vi "niDTS Comm to Comm Telnet.vi"(7 "Comm Handle":T1, 9 "error in (no error)":errorcluster) -> (8 "Comm String Handle Out":T2, 10 "error out":errorcluster)   [LabVIEW 2014, in "niDTS CommLib.lvlib"]
doc: "This sends the Command concatenated with the Args over the String Interface.\n\nInputs:\n* Command (Required): This is the command to be sent.\n* Args (Optional): Any arguments to be concatenated with the command.\n\nOutputs:\n* Response: Any data returned from the interface. Note that no data wil be returned if the flag Read Enabled is set to FALSE."
uses:
  niDTS CommLib.lvlib
  Includes/niDTS Comm String INC Handle.ctl
  Objects/String_class/niDTS Comm String.lvclass
  Framework/Comm/Includes/niDTS Comm INC Handle.ctl
  Framework/Comm/Objects/BASE_class/niDTS Comm.lvclass
  Includes/niDTS Comm Telnet INC Handle.ctl
  Objects/Telnet_class/niDTS Comm Telnet.lvclass
  Framework/niDTS Framework.lvlib
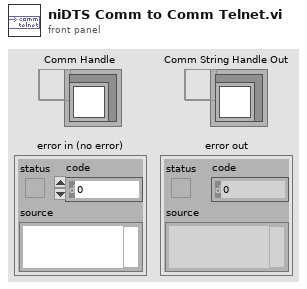
[diagram p1: front panel]
types:
  T1 = typedef "niDTS Framework.lvlib/niDTS Comm INC Handle.ctl" = refnum<data-value>
  T2 = typedef "niDTS CommLib.lvlib/niDTS Comm String INC Handle.ctl" = refnum<data-value>
  T3 = typedef "niDTS CommLib.lvlib/niDTS Comm Telnet INC Handle.ctl" = refnum<data-value>
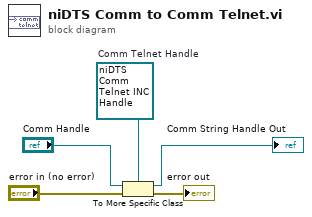
[diagram p0: block diagram]
diagram:
  w1 = T3 refnum  # Comm Telnet Handle
  n1 = To More Specific Class(target class=w1, reference="Comm Handle", error in="error in (no error)") -> (specific class reference=→"Comm String Handle Out":T3, error out=→"error out":errorcluster)
